vi "check_amplitude_sweep_parameters.vi"(8 "error in (no error)":errorcluster, 10 "Amplitude Sweep Parameters":T1={"f (Hz)"=0.0, "Number of steps"=2, "Total time (s)"=0.0, "amp_start (V)"=2000.0, "Modulation Depth (0.0 %)"=0.0, "Channel (1:Channel 1)"=2, "amp_end (V)"=2000.0, "fc (Hz)"=0.0, "DC Offset (V)"=0.0} {"DC Offset (V)" min=-20.0 max=20.0 format="%#_13g"; "fc (Hz)" min=0.0; "amp_end (V)" min=0.0 max=20.0 format="%#_13g"; "Channel (1:Channel 1)" items=["Channel 1"=1, "Channel 2"=2]; "Modulation Depth (0.0 %)" min=0.0 max=120.0 format="%.1f"; "amp_start (V)" min=0.0 max=20.0 format="%#_13g"; "Total time (s)" min=0.0; "Number of steps" min=2; "f (Hz)" min=0.0}) -> (0 "error out":errorcluster, 1 "Array":dbl[](array[numeric]), 2 "Entered Values OK":bool)   [LabVIEW 2024, in "Sweep.lvlib"]
uses:
  Sweep.lvlib
  Type Definitions/Amplitude_sweep Parameters.ctl
panel:
  out "fc (Hz)":dbl
  out "Number of frequencies":i32
  out "Total time T (s)":dbl
  out "Channel (1:Channel 1)":i32
  out "Modulation Depth (0.0 %)":dbl
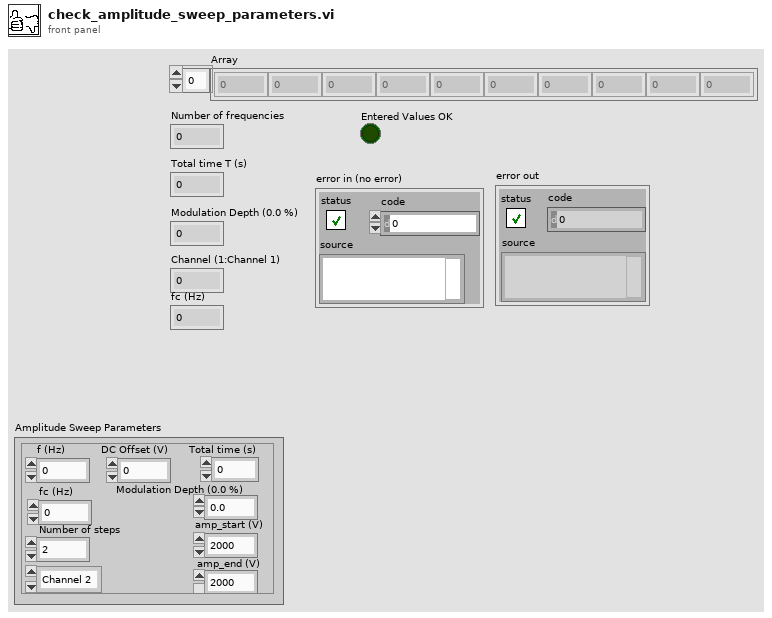
[diagram p1: front panel]
types:
  T1 = typedef "Amplitude_sweep Parameters.ctl" = cluster{"f (Hz)":dbl, "Number of steps":i32, "Total time (s)":dbl, "amp_start (V)":dbl, "Modulation Depth (0.0 %)":dbl, "Channel (1:Channel 1)":i32, "amp_end (V)":dbl, "fc (Hz)":dbl, "DC Offset (V)":dbl}
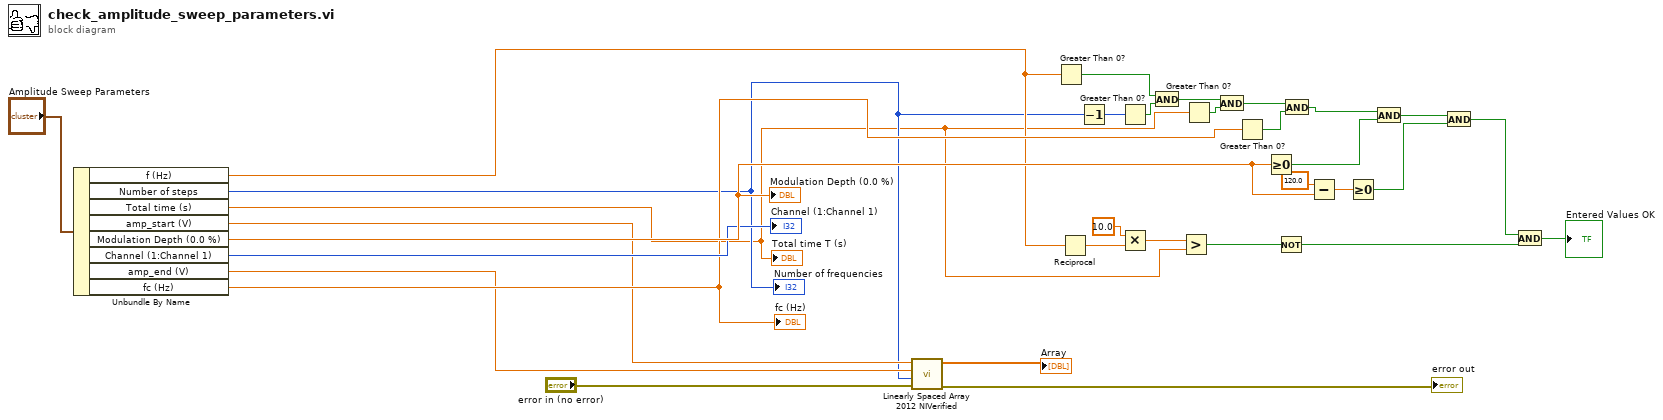
[diagram p0: block diagram]
diagram:
  n1 = Unbundle By Name("Amplitude Sweep Parameters") -> ("f (Hz)"=w3:dbl, "Number of steps"=w2:i32, "Total time (s)"=w1:dbl, "amp_start (V)"=w5:dbl, "Modulation Depth (0.0 %)"=w8:dbl, "Channel (1:Channel 1)"=→"Channel (1:Channel 1)":i32, "amp_end (V)"=w4:dbl, "fc (Hz)"=w6:dbl)
  "Modulation Depth (0.0 %)" <- w8
  "Total time T (s)" <- w1
  "Number of frequencies" <- w2
  "fc (Hz)" <- w6
  n2 = call "Linearly Spaced Array 2012 NIVerified.vi"("error in (no error)"="error in (no error)", "Number of Samples"=w2, "End"=w4, "Start"=w5) -> ("error out"=→"error out":errorcluster, "Array"=→"Array":dbl[])  [unwired: 6 in]
  n3 = Greater Than 0?(x=w3) -> (x > 0?=w23:bool)
  n4 = Reciprocal(x=w3) -> (1/x=w11:dbl)
  n5 = Decrement(x=w2) -> (x-1=w19:i32)
  n6 = Greater Than 0?(x=w19) -> (x > 0?=w24:bool)
  n7 = Multiply(x=10.0, y=w11) -> (x*y=w30:dbl)
  n8 = And(x=w23, y=w24) -> (x .and. y?=w25:bool)
  n9 = Greater?(x=w30, y=w1) -> (0:w31:bool)
  n10 = Greater Than 0?(x=w1) -> (x > 0?=w26:bool)
  n11 = And(x=w25, y=w26) -> (x .and. y?=w27:bool)
  n12 = Greater Than 0?(x=w6) -> (x > 0?=w28:bool)
  n13 = Greater Or Equal To 0?(x=w8) -> (x >= 0?=w18:bool)
  n14 = Not(x=w31) -> (.not. x?=w32:bool)
  n15 = And(x=w27, y=w28) -> (x .and. y?=w12:bool)
  n16 = Subtract(x=120.0, y=w8) -> (x-y=w15:dbl)
  n17 = Greater Or Equal To 0?(x=w15) -> (x >= 0?=w14:bool)
  n18 = And(x=w12, y=w18) -> (x .and. y?=w16:bool)
  n19 = And(x=w16, y=w14) -> (x .and. y?=w17:bool)
  n20 = And(x=w17, y=w32) -> (x .and. y?=→"Entered Values OK":bool)
